vi "cRio-IO_Lesen-Schreiben.vi"(6 "Aktion":enum16{"Eingänge lesen", "Ausgänge schreiben"}(ring), 8 "Fehler Eingang":errorcluster) -> (0 "Fehler Ausgang":errorcluster)   [LabVIEW 2020, in "Verwaltung - cRIO.lvlib"]
uses:
  Verwaltung - cRIO.lvlib
  Digital Eingaenge 0-15.ctl
  FGV IN Aktionen.ctl
  FGV OUT Aktionen.ctl
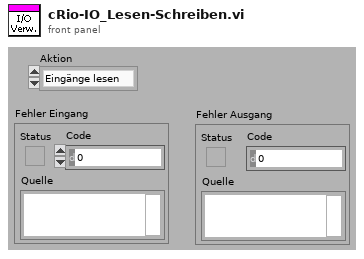
[diagram p1: front panel]
types:
  T1 = typedef "Verwaltung - cRIO.lvlib/FGV IN Aktionen.ctl" = enum16{"lesen", "DI", "AI", "Fühler Br.", "TC", "Fühler Br. TC"}
  T2 = typedef "Verwaltung - cRIO.lvlib/Digital Eingaenge 0-15.ctl" = cluster{"I0: N2 Nachf. FT-IR voll":bool, "I1: N2 Nachf. Vorrat leer":bool, "I2: (Klimaanlage eingeschaltet)":bool, "I3: (Klimaanlage Störung)":bool, "I4: Trigger Eingang (Messdaten sp.)":bool, "I5: Reserve":bool, "I6: Reserve":bool, "I7: Reserve":bool, "I8: Druckschalter Versorgung ok":bool, "I9: Reserve":bool, "I10: Reserve":bool, "I11: Reserve":bool, "I12: Drucksch. N2 Versorgung":bool, "I13: Reserve":bool, "I14: Drucksch. N2 Optikbox":bool, "I15: (Füllstand Kondensatbehälter)":bool}
  T3 = typedef "Verwaltung - cRIO.lvlib/FGV OUT Aktionen.ctl" = enum16{"lesen", "ANA OUT", "DO 0-31", "DO 32-47"}
  T4 = cluster{"Temperaturen[0]":sgl, "Temperaturen[1]":sgl, "Temperaturen[2]":sgl, "Temperaturen[3]":sgl, "Temperaturen[4]":sgl, "Temperaturen[5]":sgl, "Temperaturen[6]":sgl, "Temperaturen[7]":sgl, "Temperaturen[8]":sgl, "Temperaturen[9]":sgl, "Temperaturen[10]":sgl, "Temperaturen[11]":sgl}
  T5 = cluster{"Fühlerbruch[0]":bool, "Fühlerbruch[1]":bool, "Fühlerbruch[2]":bool, "Fühlerbruch[3]":bool, "Fühlerbruch[4]":bool, "Fühlerbruch[5]":bool, "Fühlerbruch[6]":bool, "Fühlerbruch[7]":bool, "Fühlerbruch[8]":bool, "Fühlerbruch[9]":bool, "Fühlerbruch[10]":bool, "Fühlerbruch[11]":bool}
  T6 = cluster{"Fühlerbruch[0]":bool, "Fühlerbruch[1]":bool, "Fühlerbruch[2]":bool, "Fühlerbruch[3]":bool, "Fühlerbruch[4]":bool, "Fühlerbruch[5]":bool, "Fühlerbruch[6]":bool, "Fühlerbruch[7]":bool}
  T7 = cluster{"[0]":sgl, "[1]":sgl, "[2]":sgl, "[3]":sgl, "[4]":sgl, "[5]":sgl, "[6]":sgl, "[7]":sgl, "[8]":sgl, "[9]":sgl, "[10]":sgl, "[11]":sgl, "[12]":sgl, "[13]":sgl, "[14]":sgl, "[15]":sgl, "[16]":sgl}
  T8 = typedef "Verwaltung - cRIO.lvlib/Digital Ausgaenge 0-31.ctl" = cluster{"O0: Druckluft Versorgung":bool, "O1: CG 1 (FB Eingang 1)":bool, "O2: CG 2 (Kühlung FT-IR EIN)":bool, "O3: CG 3 (FB Bypass)":bool, "O4: CG 4 (FB CalGas)":bool, "O5: CG 5 (FB spülen/UL)":bool, "O6: CG 6 (FB zum FT-IR)":bool, "O7: CG 7 (FB zum FID)":bool, "O8: CG 8 (FB Reserve)":bool, "O9: (FB Reserve)":bool, "O10: (FB Umgebungsluft FID)":bool, "O11: (FB zum Gaskühler)":bool, "O12: FB Stickstoff zu FT-IR":bool, "O13: Optikbox FT-IR spülen":bool, "O14: (Purifier deaktivieren)":bool, "O15: (Umschaltung Purifier/Stickstoff)":bool, "O16: N2 Einblasung":bool, "O17: LSP LN2 Nachfüllung":bool, "O18: (Reserve)":bool, "O19: (Pumpe Eingang1)":bool, "O20: (Pumpe Eingang2)":bool, "O21: (Pumpe Spülen1)":bool, "O22: (Pumpe Spülen2)":bool, "O23: (Reserve)":bool, "O24: CalGas 1":bool, "O25: CalGas 2":bool, "O26: CG 3-8 (CalGas 3)":bool, "O27: Stickstoff aufschalten":bool, "O28: CG zu PNS":bool, "O29: FTIR Standby Spülung":bool, "O30: CG zu Entnahme(T90)":bool, "O31: (Purifier regenerieren)":bool}
  T9 = typedef "Verwaltung - cRIO.lvlib/Digital Ausgaenge 32-63.ctl" = cluster{"O32: Messgaspumpe EIN":bool, "O33: (Umgebungsluftpumpe)":bool, "O34: (Kondensatpumpe GK)":bool, "O35: Klima/Lüfter EIN":bool, "O36: Versorgung Heizungen":bool, "O37: Versorgung Heizungen":bool, "O38: (Gaskühler EIN (Freigabe))":bool, "O39: Störung FAS LP":bool, "O40: (Heizung Filterblock)":bool, "O41: Heizung HL zu FT-IR":bool, "O42: Heizung HL Extern SP1":bool, "O43: Heizung HL Extern SP2":bool, "O44: Heizung Reserve":bool, "O45: Heizung Reserve":bool, "O46: Statusbeleuchtung grün":bool, "O47: Statusbeleuchtung rot":bool}
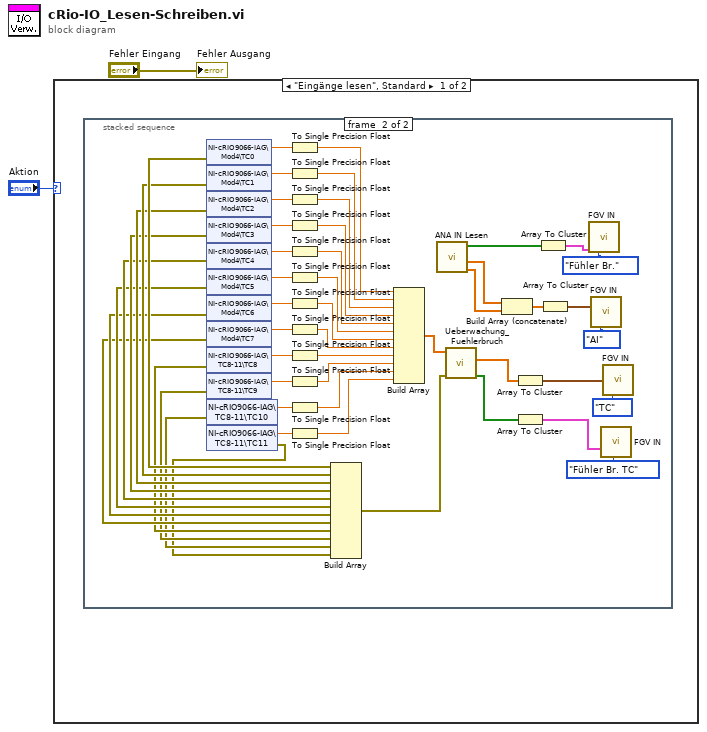
[diagram p0: block diagram]
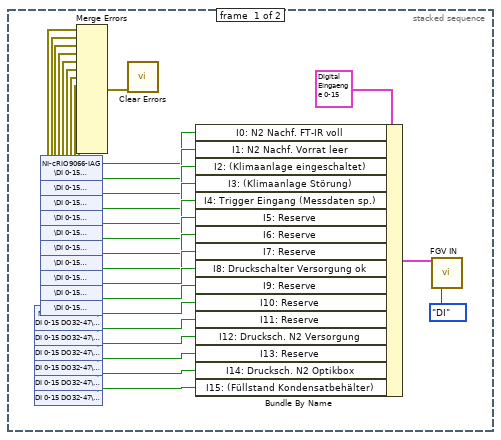
[diagram p2: hidden frame]
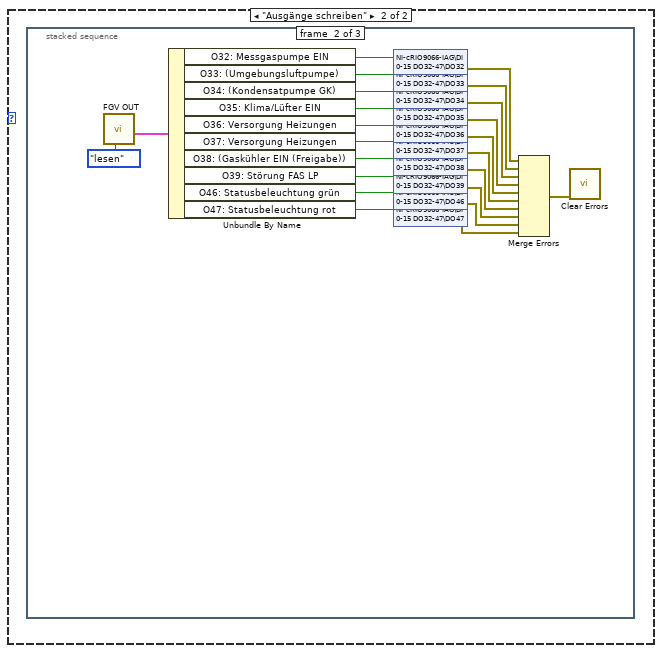
[diagram p3: hidden frame]
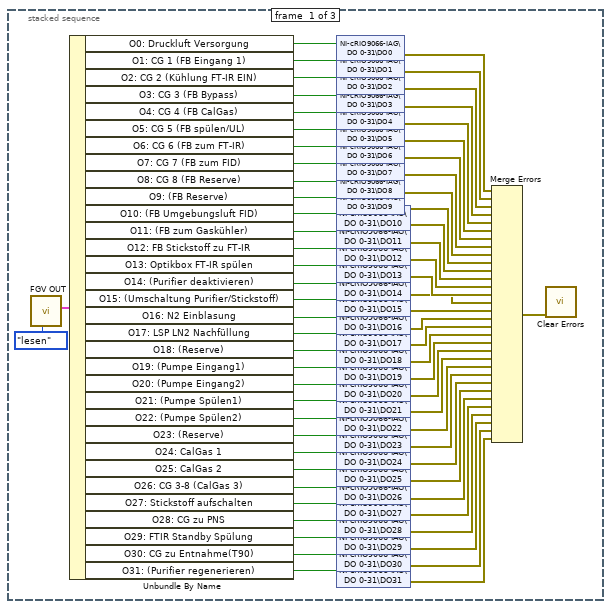
[diagram p4: hidden frame]
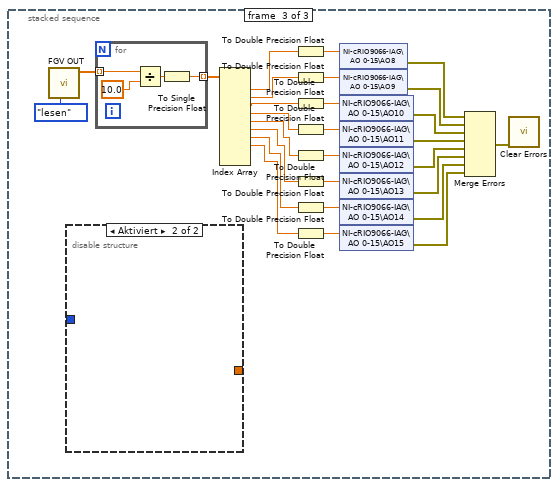
[diagram p5: hidden frame]
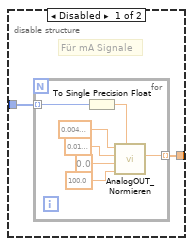
[diagram p6: hidden frame]
diagram:
  n1 = case shown="\"Eingänge lesen\", Standard" "Aktion" {
    frame "Eingänge lesen", Default {
      n2 = stacked-sequence {
        frame #0 {
          n3 = shared-variable "NI-cRIO9066-IAG\\DI 0-15 DO32-47\\DI10"() -> (w34:bool, error out=w10:errorcluster)  [unwired: 1 out]
          n4 = shared-variable "NI-cRIO9066-IAG\\DI 0-15 DO32-47\\DI11"() -> (w37:bool, error out=w9:errorcluster)  [unwired: 1 out]
          n5 = shared-variable "NI-cRIO9066-IAG\\DI 0-15 DO32-47\\DI12"() -> (w38:bool, error out=w8:errorcluster)  [unwired: 1 out]
          n6 = shared-variable "NI-cRIO9066-IAG\\DI 0-15 DO32-47\\DI13"() -> (w36:bool, error out=w7:errorcluster)  [unwired: 1 out]
          n7 = shared-variable "NI-cRIO9066-IAG\\DI 0-15 DO32-47\\DI14"() -> (w22:bool, error out=w6:errorcluster)  [unwired: 1 out]
          n8 = shared-variable "NI-cRIO9066-IAG\\DI 0-15 DO32-47\\DI15"() -> (w35:bool, error out=w5:errorcluster)  [unwired: 1 out]
          n9 = shared-variable "NI-cRIO9066-IAG\\DI 0-15 DO32-47\\DI0"() -> (w24:bool, error out=w20:errorcluster)  [unwired: 1 out]
          n10 = shared-variable "NI-cRIO9066-IAG\\DI 0-15 DO32-47\\DI1"() -> (w25:bool, error out=w19:errorcluster)  [unwired: 1 out]
          n11 = shared-variable "NI-cRIO9066-IAG\\DI 0-15 DO32-47\\DI2"() -> (w26:bool, error out=w18:errorcluster)  [unwired: 1 out]
          n12 = shared-variable "NI-cRIO9066-IAG\\DI 0-15 DO32-47\\DI3"() -> (w27:bool, error out=w17:errorcluster)  [unwired: 1 out]
          n13 = shared-variable "NI-cRIO9066-IAG\\DI 0-15 DO32-47\\DI4"() -> (w28:bool, error out=w16:errorcluster)  [unwired: 1 out]
          n14 = shared-variable "NI-cRIO9066-IAG\\DI 0-15 DO32-47\\DI5"() -> (w29:bool, error out=w15:errorcluster)  [unwired: 1 out]
          n15 = shared-variable "NI-cRIO9066-IAG\\DI 0-15 DO32-47\\DI6"() -> (w30:bool, error out=w14:errorcluster)  [unwired: 1 out]
          n16 = shared-variable "NI-cRIO9066-IAG\\DI 0-15 DO32-47\\DI7"() -> (w31:bool, error out=w13:errorcluster)  [unwired: 1 out]
          n17 = shared-variable "NI-cRIO9066-IAG\\DI 0-15 DO32-47\\DI8"() -> (w32:bool, error out=w12:errorcluster)  [unwired: 1 out]
          n18 = shared-variable "NI-cRIO9066-IAG\\DI 0-15 DO32-47\\DI9"() -> (w33:bool, error out=w11:errorcluster)  [unwired: 1 out]
          n19 = Merge Errors(w20, w19, w18, w17, w16, w15, w14, w13, w12, w11, w10, w9, w8, w7, w6, w5) -> (w21:errorcluster)
          n20 = call <vilib>:"Clear Errors.vi"("error in (no error)"=w21) -> ()  [unwired: 5 in, 2 out]
          n21 = Bundle By Name(cluster=T2 {"I0: N2 Nachf. FT-IR voll"=FALSE, "I1: N2 Nachf. Vorrat leer"=FALSE, "I2: (Klimaanlage eingeschaltet)"=FALSE, "I3: (Klimaanlage Störung)"=FALSE, "I4: Trigger Eingang (Messdaten sp.)"=FALSE, "I5: Reserve"=FALSE, "I6: Reserve"=FALSE, "I7: Reserve"=FALSE, "I8: Druckschalter Versorgung ok"=FALSE, "I9: Reserve"=FALSE, "I10: Reserve"=FALSE, "I11: Reserve"=FALSE, "I12: Drucksch. N2 Versorgung"=FALSE, "I13: Reserve"=FALSE, "I14: Drucksch. N2 Optikbox"=FALSE, "I15: (Füllstand Kondensatbehälter)"=FALSE} ("DI"), "I0: N2 Nachf. FT-IR voll"=w24, "I1: N2 Nachf. Vorrat leer"=w25, "I2: (Klimaanlage eingeschaltet)"=w26, "I3: (Klimaanlage Störung)"=w27, "I4: Trigger Eingang (Messdaten sp.)"=w28, "I5: Reserve"=w29, "I6: Reserve"=w30, "I7: Reserve"=w31, "I8: Druckschalter Versorgung ok"=w32, "I9: Reserve"=w33, "I10: Reserve"=w34, "I11: Reserve"=w37, "I12: Drucksch. N2 Versorgung"=w38, "I13: Reserve"=w36, "I14: Drucksch. N2 Optikbox"=w22, "I15: (Füllstand Kondensatbehälter)"=w35) -> (w3:T2)
          n22 = call "FGV IN.vi"("DI"=w3, "Aktion"=FGV_IN_Aktionen."DI") -> ()  [unwired: 9 in, 5 out]
        }
        frame #1 {
          n23 = shared-variable "NI-cRIO9066-IAG\\Mod4\\TC0"() -> (w83:dbl, error out=w69:errorcluster)  [unwired: 1 in]
          n24 = shared-variable "NI-cRIO9066-IAG\\Mod4\\TC1"() -> (w90:dbl, error out=w68:errorcluster)  [unwired: 1 in]
          n25 = shared-variable "NI-cRIO9066-IAG\\Mod4\\TC2"() -> (w89:dbl, error out=w67:errorcluster)  [unwired: 1 in]
          n26 = shared-variable "NI-cRIO9066-IAG\\Mod4\\TC3"() -> (w88:dbl, error out=w66:errorcluster)  [unwired: 1 in]
          n27 = shared-variable "NI-cRIO9066-IAG\\Mod4\\TC4"() -> (w87:dbl, error out=w65:errorcluster)  [unwired: 1 in]
          n28 = shared-variable "NI-cRIO9066-IAG\\Mod4\\TC5"() -> (w86:dbl, error out=w64:errorcluster)  [unwired: 1 in]
          n29 = shared-variable "NI-cRIO9066-IAG\\Mod4\\TC6"() -> (w85:dbl, error out=w63:errorcluster)  [unwired: 1 in]
          n30 = shared-variable "NI-cRIO9066-IAG\\Mod4\\TC7"() -> (w84:dbl, error out=w62:errorcluster)  [unwired: 1 in]
          n31 = shared-variable "NI-cRIO9066-IAG\\TC8-11\\TC8"() -> (w50:dbl, error out=w46:errorcluster)  [unwired: 1 in]
          n32 = shared-variable "NI-cRIO9066-IAG\\TC8-11\\TC9"() -> (w49:dbl, error out=w45:errorcluster)  [unwired: 1 in]
          n33 = shared-variable "NI-cRIO9066-IAG\\TC8-11\\TC10"() -> (w48:dbl, error out=w44:errorcluster)  [unwired: 1 in]
          n34 = shared-variable "NI-cRIO9066-IAG\\TC8-11\\TC11"() -> (w47:dbl, error out=w43:errorcluster)  [unwired: 1 in]
          n35 = To Single Precision Float(number=w83) -> (single precision float=w79:sgl)
          n36 = To Single Precision Float(number=w90) -> (single precision float=w75:sgl)
          n37 = To Single Precision Float(number=w89) -> (single precision float=w74:sgl)
          n38 = To Single Precision Float(number=w88) -> (single precision float=w73:sgl)
          n39 = To Single Precision Float(number=w87) -> (single precision float=w72:sgl)
          n40 = To Single Precision Float(number=w86) -> (single precision float=w76:sgl)
          n41 = To Single Precision Float(number=w85) -> (single precision float=w77:sgl)
          n42 = To Single Precision Float(number=w84) -> (single precision float=w78:sgl)
          n43 = To Single Precision Float(number=w50) -> (single precision float=w42:sgl)
          n44 = To Single Precision Float(number=w49) -> (single precision float=w41:sgl)
          n45 = To Single Precision Float(number=w48) -> (single precision float=w40:sgl)
          n46 = To Single Precision Float(number=w47) -> (single precision float=w39:sgl)
          n47 = Build Array(w69, w68, w67, w66, w65, w64, w63, w62, w46, w45, w44, w43) -> (w61:errorcluster[])
          n48 = Build Array(w79, w75, w74, w73, w72, w76, w77, w78, w42, w41, w40, w39) -> (w80:sgl[])
          n49 = call "ANA IN Lesen.vi"() -> ("Rohwerte"=w54:sgl[], "Istwerte"=w82:sgl[], "Fühlerbruch"=w51:bool[])  [unwired: 9 in]
          n50 = call "Ueberwachung_Fuehlerbruch.vi"("Angehängtes Array"=w61, "AI - TC Eingang"=w80) -> ("Fühlerbruch"=w55:bool[], "Temperaturen"=w59:sgl[])  [unwired: 2 in, 6 out]
          n51 = Build Array (concatenate)(w82, w54) -> (w81:sgl[])
          n52 = Array To Cluster(array=w59) -> (cluster=w58:T4)
          n53 = Array To Cluster(array=w55) -> (cluster=w56:T5)
          n54 = Array To Cluster(array=w51) -> (cluster=w52:T6)
          n55 = Array To Cluster(array=w81) -> (cluster=w53:T7)
          n56 = call "FGV IN.vi"("Fühler Bruch AI"=w52, "Aktion"=FGV_IN_Aktionen."Fühler Br.") -> ()  [unwired: 9 in, 5 out]
          n57 = call "FGV IN.vi"("Analog Eingänge"=w53, "Aktion"=FGV_IN_Aktionen."AI") -> ()  [unwired: 9 in, 5 out]
          n58 = call "FGV IN.vi"("Fühler Bruch TC"=w56, "Aktion"=FGV_IN_Aktionen."Fühler Br. TC") -> ()  [unwired: 9 in, 5 out]
          n59 = call "FGV IN.vi"("TC Eingänge"=w58, "Aktion"=FGV_IN_Aktionen."TC") -> ()  [unwired: 9 in, 5 out]
        }
      }
    }
    frame "Ausgänge schreiben" {
      n60 = stacked-sequence {
        frame #0 {
          n61 = call "FGV OUT.vi"("Aktion"=FGV_OUT_Aktionen."lesen") -> ("DO 0-31"=w91:T8)  [unwired: 7 in, 3 out]
          n62 = Unbundle By Name(w91) -> ("O0: Druckluft Versorgung"=w137:bool, "O1: CG 1 (FB Eingang 1)"=w138:bool, "O2: CG 2 (Kühlung FT-IR EIN)"=w139:bool, "O3: CG 3 (FB Bypass)"=w140:bool, "O4: CG 4 (FB CalGas)"=w141:bool, "O5: CG 5 (FB spülen/UL)"=w142:bool, "O6: CG 6 (FB zum FT-IR)"=w143:bool, "O7: CG 7 (FB zum FID)"=w144:bool, "O8: CG 8 (FB Reserve)"=w145:bool, "O9: (FB Reserve)"=w146:bool, "O10: (FB Umgebungsluft FID)"=w147:bool, "O11: (FB zum Gaskühler)"=w148:bool, "O12: FB Stickstoff zu FT-IR"=w149:bool, "O13: Optikbox FT-IR spülen"=w150:bool, "O14: (Purifier deaktivieren)"=w157:bool, "O15: (Umschaltung Purifier/Stickstoff)"=w132:bool, "O16: N2 Einblasung"=w156:bool, "O17: LSP LN2 Nachfüllung"=w155:bool, "O18: (Reserve)"=w154:bool, "O19: (Pumpe Eingang1)"=w135:bool, "O20: (Pumpe Eingang2)"=w134:bool, "O21: (Pumpe Spülen1)"=w131:bool, "O22: (Pumpe Spülen2)"=w130:bool, "O23: (Reserve)"=w129:bool, "O24: CalGas 1"=w128:bool, "O25: CalGas 2"=w127:bool, "O26: CG 3-8 (CalGas 3)"=w126:bool, "O27: Stickstoff aufschalten"=w136:bool, "O28: CG zu PNS"=w153:bool, "O29: FTIR Standby Spülung"=w152:bool, "O30: CG zu Entnahme(T90)"=w133:bool, "O31: (Purifier regenerieren)"=w151:bool)
          n63 = shared-variable "NI-cRIO9066-IAG\\DO 0-31\\DO0"(w137) -> (error out=w125:errorcluster)  [unwired: 1 out]
          n64 = shared-variable "NI-cRIO9066-IAG\\DO 0-31\\DO1"(w138) -> (error out=w124:errorcluster)  [unwired: 1 out]
          n65 = shared-variable "NI-cRIO9066-IAG\\DO 0-31\\DO2"(w139) -> (error out=w123:errorcluster)  [unwired: 1 out]
          n66 = shared-variable "NI-cRIO9066-IAG\\DO 0-31\\DO3"(w140) -> (error out=w122:errorcluster)  [unwired: 1 out]
          n67 = shared-variable "NI-cRIO9066-IAG\\DO 0-31\\DO4"(w141) -> (error out=w121:errorcluster)  [unwired: 1 out]
          n68 = shared-variable "NI-cRIO9066-IAG\\DO 0-31\\DO5"(w142) -> (error out=w120:errorcluster)  [unwired: 1 out]
          n69 = shared-variable "NI-cRIO9066-IAG\\DO 0-31\\DO6"(w143) -> (error out=w119:errorcluster)  [unwired: 1 out]
          n70 = shared-variable "NI-cRIO9066-IAG\\DO 0-31\\DO7"(w144) -> (error out=w118:errorcluster)  [unwired: 1 out]
          n71 = shared-variable "NI-cRIO9066-IAG\\DO 0-31\\DO8"(w145) -> (error out=w117:errorcluster)  [unwired: 1 out]
          n72 = shared-variable "NI-cRIO9066-IAG\\DO 0-31\\DO9"(w146) -> (error out=w116:errorcluster)  [unwired: 1 out]
          n73 = shared-variable "NI-cRIO9066-IAG\\DO 0-31\\DO10"(w147) -> (error out=w115:errorcluster)  [unwired: 1 out]
          n74 = shared-variable "NI-cRIO9066-IAG\\DO 0-31\\DO11"(w148) -> (error out=w114:errorcluster)  [unwired: 1 out]
          n75 = shared-variable "NI-cRIO9066-IAG\\DO 0-31\\DO12"(w149) -> (error out=w113:errorcluster)  [unwired: 1 out]
          n76 = shared-variable "NI-cRIO9066-IAG\\DO 0-31\\DO13"(w150) -> (error out=w112:errorcluster)  [unwired: 1 out]
          n77 = shared-variable "NI-cRIO9066-IAG\\DO 0-31\\DO14"(w157) -> (error out=w111:errorcluster)  [unwired: 1 out]
          n78 = shared-variable "NI-cRIO9066-IAG\\DO 0-31\\DO15"(w132) -> (error out=w110:errorcluster)  [unwired: 1 in]
          n79 = shared-variable "NI-cRIO9066-IAG\\DO 0-31\\DO16"(w156) -> (error out=w109:errorcluster)  [unwired: 1 out]
          n80 = shared-variable "NI-cRIO9066-IAG\\DO 0-31\\DO17"(w155) -> (error out=w108:errorcluster)  [unwired: 1 out]
          n81 = shared-variable "NI-cRIO9066-IAG\\DO 0-31\\DO18"(w154) -> (error out=w107:errorcluster)  [unwired: 1 out]
          n82 = shared-variable "NI-cRIO9066-IAG\\DO 0-31\\DO19"(w135) -> (error out=w106:errorcluster)  [unwired: 1 out]
          n83 = shared-variable "NI-cRIO9066-IAG\\DO 0-31\\DO20"(w134) -> (error out=w105:errorcluster)  [unwired: 1 in]
          n84 = shared-variable "NI-cRIO9066-IAG\\DO 0-31\\DO21"(w131) -> (error out=w104:errorcluster)  [unwired: 1 in]
          n85 = shared-variable "NI-cRIO9066-IAG\\DO 0-31\\DO22"(w130) -> (error out=w103:errorcluster)  [unwired: 1 in]
          n86 = shared-variable "NI-cRIO9066-IAG\\DO 0-31\\DO23"(w129) -> (error out=w102:errorcluster)  [unwired: 1 in]
          n87 = shared-variable "NI-cRIO9066-IAG\\DO 0-31\\DO24"(w128) -> (error out=w101:errorcluster)  [unwired: 1 in]
          n88 = shared-variable "NI-cRIO9066-IAG\\DO 0-31\\DO25"(w127) -> (error out=w100:errorcluster)  [unwired: 1 in]
          n89 = shared-variable "NI-cRIO9066-IAG\\DO 0-31\\DO26"(w126) -> (error out=w99:errorcluster)  [unwired: 1 in]
          n90 = shared-variable "NI-cRIO9066-IAG\\DO 0-31\\DO27"(w136) -> (error out=w98:errorcluster)  [unwired: 1 out]
          n91 = shared-variable "NI-cRIO9066-IAG\\DO 0-31\\DO28"(w153) -> (error out=w97:errorcluster)  [unwired: 1 out]
          n92 = shared-variable "NI-cRIO9066-IAG\\DO 0-31\\DO29"(w152) -> (error out=w96:errorcluster)  [unwired: 1 out]
          n93 = shared-variable "NI-cRIO9066-IAG\\DO 0-31\\DO30"(w133) -> (error out=w95:errorcluster)  [unwired: 1 in]
          n94 = shared-variable "NI-cRIO9066-IAG\\DO 0-31\\DO31"(w151) -> (error out=w94:errorcluster)  [unwired: 1 out]
          n95 = Merge Errors(w125, w124, w123, w122, w121, w120, w119, w118, w117, w116, w115, w114, w113, w112, w111, w110, w109, w108, w107, w106, w105, w104, w103, w102, w101, w100, w99, w98, w97, w96, w95, w94) -> (w93:errorcluster)
          n96 = call <vilib>:"Clear Errors.vi"("error in (no error)"=w93) -> ()  [unwired: 5 in, 2 out]
        }
        frame #1 {
          n97 = call "FGV OUT.vi"("Aktion"=FGV_OUT_Aktionen."lesen") -> ("DO 32-63"=w163:T9)  [unwired: 7 in, 3 out]
          n98 = Unbundle By Name(w163) -> ("O32: Messgaspumpe EIN"=w174:bool, "O33: (Umgebungsluftpumpe)"=w175:bool, "O34: (Kondensatpumpe GK)"=w176:bool, "O35: Klima/Lüfter EIN"=w177:bool, "O36: Versorgung Heizungen"=w178:bool, "O37: Versorgung Heizungen"=w179:bool, "O38: (Gaskühler EIN (Freigabe))"=w162:bool, "O39: Störung FAS LP"=w180:bool, "O46: Statusbeleuchtung grün"=w161:bool, "O47: Statusbeleuchtung rot"=w160:bool)
          n99 = shared-variable "NI-cRIO9066-IAG\\DI 0-15 DO32-47\\DO32"(w174) -> (error out=w172:errorcluster)  [unwired: 1 in]
          n100 = shared-variable "NI-cRIO9066-IAG\\DI 0-15 DO32-47\\DO33"(w175) -> (error out=w171:errorcluster)  [unwired: 1 in]
          n101 = shared-variable "NI-cRIO9066-IAG\\DI 0-15 DO32-47\\DO34"(w176) -> (error out=w170:errorcluster)  [unwired: 1 in]
          n102 = shared-variable "NI-cRIO9066-IAG\\DI 0-15 DO32-47\\DO35"(w177) -> (error out=w169:errorcluster)  [unwired: 1 in]
          n103 = shared-variable "NI-cRIO9066-IAG\\DI 0-15 DO32-47\\DO36"(w178) -> (error out=w168:errorcluster)  [unwired: 1 in]
          n104 = shared-variable "NI-cRIO9066-IAG\\DI 0-15 DO32-47\\DO37"(w179) -> (error out=w167:errorcluster)  [unwired: 1 in]
          n105 = shared-variable "NI-cRIO9066-IAG\\DI 0-15 DO32-47\\DO38"(w162) -> (error out=w166:errorcluster)  [unwired: 1 in]
          n106 = shared-variable "NI-cRIO9066-IAG\\DI 0-15 DO32-47\\DO39"(w180) -> (error out=w165:errorcluster)  [unwired: 1 in]
          n107 = shared-variable "NI-cRIO9066-IAG\\DI 0-15 DO32-47\\DO46"(w161) -> (error out=w159:errorcluster)  [unwired: 1 in]
          n108 = shared-variable "NI-cRIO9066-IAG\\DI 0-15 DO32-47\\DO47"(w160) -> (error out=w158:errorcluster)  [unwired: 1 in]
          n109 = Merge Errors(w172, w171, w170, w169, w168, w167, w166, w165, w159, w158) -> (w173:errorcluster)
          n110 = call <vilib>:"Clear Errors.vi"("error in (no error)"=w173) -> ()  [unwired: 5 in, 2 out]
        }
        frame #2 {
          n111 = call "FGV OUT.vi"("Aktion"=FGV_OUT_Aktionen."lesen") -> ("ANA OUT"=w189:sgl[])  [unwired: 7 in, 3 out]
          n112 = disable-structure shown="Aktiviert" {
            disable-tunnel: _ -> [w214 _]
            disable-tunnel: [w213 _] -> _
            frame Disabled {
              # "Für mA Signale"
              n113 = for {
                tunnel: w214 -> [w221] mode=indexing
                tunnel: [w215] -> w213 mode=indexing
                n114 = To Single Precision Float(number=w221) -> (single precision float=w220:sgl)
                n115 = call "AnalogOUT_Normieren.vi"("Analogwert"=w220, "Obergrenze"=sgl 100.0, "Untergrenze"=sgl 0.0, "Max Analogwert"=sgl 0.02, "Min Analogwert"=sgl 0.004) -> ("Normierter Wert"=w215:sgl)  [unwired: 6 in]
              }
            }
            frame Enabled {
            }
          }
          n116 = for {
            tunnel: w189 -> [w212] mode=indexing
            tunnel: [w209] -> w208 mode=indexing
            n117 = Divide(x=w212, y=sgl 10.0) -> (x/y=w210:sgl)
            n118 = To Single Precision Float(number=w210) -> (single precision float=w209:sgl)
          }
          n119 = Index Array(array=w208) -> (element #1=w188:sgl, element #2=w187:sgl, element #3=w186:sgl, element #4=w185:sgl, element #5=w184:sgl, element #6=w183:sgl, element #7=w182:sgl, element #8=w181:sgl)  [unwired: 10 in, 2 out]
          n120 = To Double Precision Float(number=w188) -> (double precision float=w207:dbl)
          n121 = To Double Precision Float(number=w187) -> (double precision float=w206:dbl)
          n122 = To Double Precision Float(number=w186) -> (double precision float=w205:dbl)
          n123 = To Double Precision Float(number=w185) -> (double precision float=w204:dbl)
          n124 = To Double Precision Float(number=w184) -> (double precision float=w203:dbl)
          n125 = To Double Precision Float(number=w183) -> (double precision float=w202:dbl)
          n126 = To Double Precision Float(number=w182) -> (double precision float=w201:dbl)
          n127 = To Double Precision Float(number=w181) -> (double precision float=w200:dbl)
          n128 = shared-variable "NI-cRIO9066-IAG\\AO 0-15\\AO8"(w207) -> (error out=w198:errorcluster)  [unwired: 1 in]
          n129 = shared-variable "NI-cRIO9066-IAG\\AO 0-15\\AO9"(w206) -> (error out=w197:errorcluster)  [unwired: 1 in]
          n130 = shared-variable "NI-cRIO9066-IAG\\AO 0-15\\AO10"(w205) -> (error out=w196:errorcluster)  [unwired: 1 in]
          n131 = shared-variable "NI-cRIO9066-IAG\\AO 0-15\\AO11"(w204) -> (error out=w195:errorcluster)  [unwired: 1 in]
          n132 = shared-variable "NI-cRIO9066-IAG\\AO 0-15\\AO12"(w203) -> (error out=w194:errorcluster)  [unwired: 1 in]
          n133 = shared-variable "NI-cRIO9066-IAG\\AO 0-15\\AO13"(w202) -> (error out=w193:errorcluster)  [unwired: 1 in]
          n134 = shared-variable "NI-cRIO9066-IAG\\AO 0-15\\AO14"(w201) -> (error out=w192:errorcluster)  [unwired: 1 in]
          n135 = shared-variable "NI-cRIO9066-IAG\\AO 0-15\\AO15"(w200) -> (error out=w191:errorcluster)  [unwired: 1 in]
          n136 = Merge Errors(w198, w197, w196, w195, w194, w193, w192, w191) -> (w199:errorcluster)
          n137 = call <vilib>:"Clear Errors.vi"("error in (no error)"=w199) -> ()  [unwired: 5 in, 2 out]
        }
      }
    }
  }
  "Fehler Ausgang" <- "Fehler Eingang"
